vi "CalcZoomedPic.vi"(0 "Image Data In":T1, 5 "Pict Refnum":refnum<vi>, 7 "OriginPoint":T2, 9 "ZoomFactor":dbl, 11 "error in (no error)":errorcluster) -> (4 "Image Data Out":T1, 15 "error out":errorcluster)   [LabVIEW 2019, in "AnimatorXControl.xctl"]
uses:
  AnimatorXControl.xctl
  <vilib>/Utility/miscctls.llb/LVPointTypeDef.ctl
  <vilib>/picture/picture.llb/imagedata.ctl
panel:
  out "Picture":picture
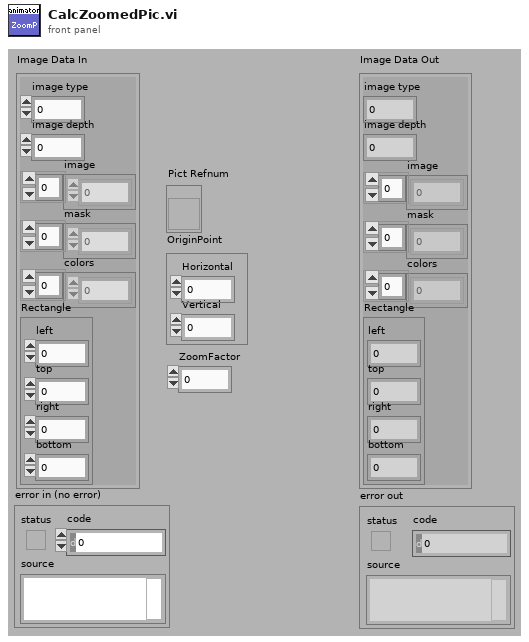
[diagram p1: front panel]
types:
  T1 = typedef "imagedata.ctl" = cluster{"image type":i32, "image depth":i32, "image":u8[], "mask":u8[], "colors":u32[], "Rectangle":cluster{"left":i16, "top":i16, "right":i16, "bottom":i16}}
  T2 = typedef "LVPointTypeDef.ctl" = cluster{"Horizontal":i16, "Vertical":i16}
  T3 = typedef "LVBoundsTypeDef.ctl" = cluster{"Width":u32, "Height":u32}
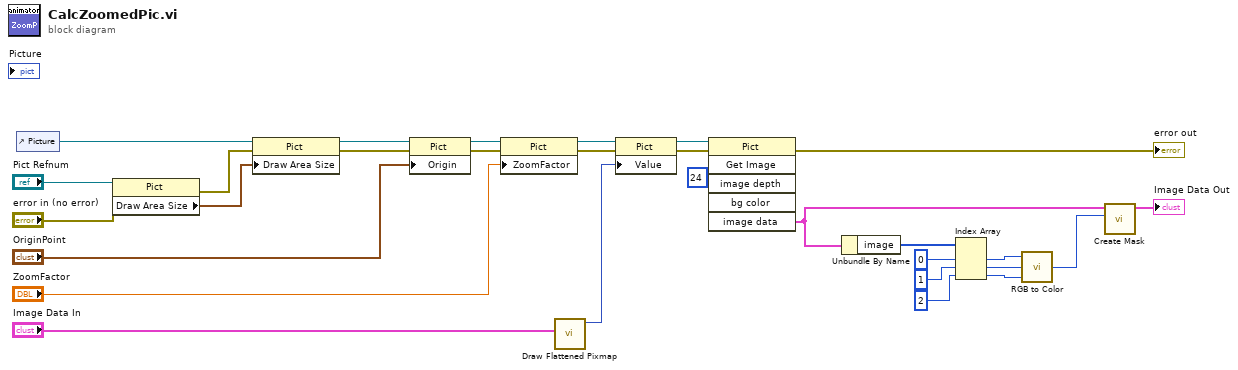
[diagram p0: block diagram]
diagram:
  n1 = control-ref of="Picture"() -> (w8:refnum<vi>)
  n2 = property class="Pict"(reference="Pict Refnum", error in="error in (no error)") -> (error out=w7:errorcluster, "Draw Area Size"=w11:T3)  [unwired: 1 out]
  n3 = property class="Pict"(reference=w8, error in=w7, "Draw Area Size"=w11) -> (reference out=w10:refnum<vi>, error out=w9:errorcluster)
  n4 = property class="Pict"(reference=w10, error in=w9, "Origin"="OriginPoint") -> (reference out=w29:refnum<vi>, error out=w28:errorcluster)
  n5 = property class="Pict"(reference=w29, error in=w28, "ZoomFactor"="ZoomFactor") -> (reference out=w27:refnum<vi>, error out=w26:errorcluster)
  n6 = call <vilib>:"Draw Flattened Pixmap.vi"("image data"="Image Data In") -> ("new picture"=w25:picture)  [unwired: 8 in]
  n7 = property class="Pict"(reference=w27, error in=w26, "Value"=w25) -> (reference out=w24:refnum<vi>, error out=w23:errorcluster)
  n8 = invoke class="Pict" method="Get Image"(reference=w24, error in=w23, "image depth"=24 ("Image Depth")) -> (error out=→"error out":errorcluster, "image data"=w17:T1)  [unwired: 3 in, 4 out]
  n9 = Unbundle By Name(w17) -> ("image"=w19:u8[])
  n10 = Index Array(array=w19, index #1=0 ("index"), index #2=1 ("index"), index #3=2 ("index")) -> (element #1=w13:u8, element #2=w4:u8, element #3=w3:u8)
  n11 = call <vilib>:"RGB to Color.vi"("B"=w3, "G"=w4, "R"=w13) -> ("Color"=w18:u32)
  n12 = call <vilib>:"Create Mask.vi"("Mask Color (Black)"=w18, "image data"=w17) -> ("image data"=→"Image Data Out":T1)  [unwired: 9 in]
